vi "byte_array_to_bool_array_setup.vi"() -> (0 "error out":errorcluster, 2 "unsigned byte array":u8[](array[numeric]))   [LabVIEW 2018]
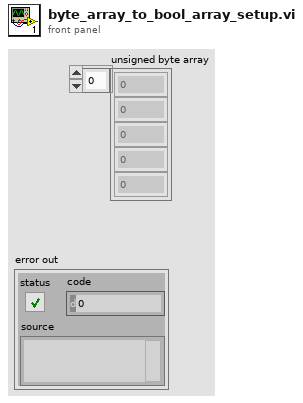
[diagram p1: front panel]
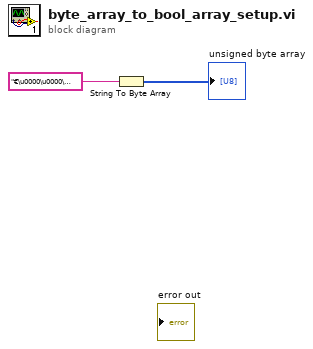
[diagram p0: block diagram]
diagram:
  n1 = String To Byte Array(string="€\u0000\u0000\u0000€" ("String")) -> (unsigned byte array=→"unsigned byte array":u8[])
